vi "FXP Read base - CAR 397265.vi"(8 "error in (no error)":errorcluster, 9 "data in":dbl, 10 "integersize":i32, 11 "shared variable refnum in":refnum<k21>) -> (0 "error out":errorcluster, 1 "data out":dbl, 3 "shared variable refnum out":refnum<k21>)   [LabVIEW 2020]
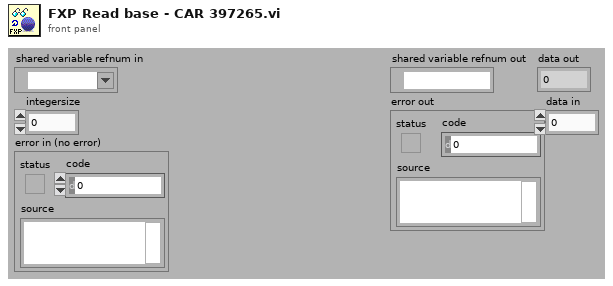
[diagram p1: front panel]
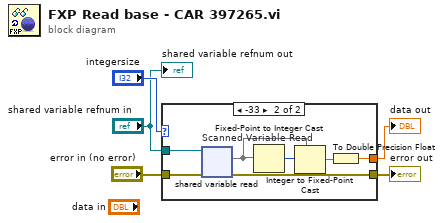
[diagram p0: block diagram]
diagram:
  n1 = case shown="-33" "integersize" {
    tunnel: "error in (no error)" -> [w6 w13]
    tunnel: [w6 w12] -> w3
    tunnel: "shared variable refnum in" -> [_ w11]
    tunnel: [_ w10] -> w1
    frame 2048, Default {
    }
    frame -33 {
      n2 = shared-variable-read "Scanned Variable Read"(w11, w13) -> (w12:errorcluster, w7)  [unwired: 1 in, 2 out]
      n3 = Fixed-Point to Integer Cast(1:w7) -> (0:w8:i32)
      n4 = Integer to Fixed-Point Cast(fixed-point type=w7, integer=w8) -> (fixed-point=w9:fxp<+/-,32,32>)
      n5 = To Double Precision Float(number=w9) -> (double precision float=w10:dbl)
    }
  }
  "error out" <- w3
  "data out" <- w1
  "shared variable refnum out" <- "shared variable refnum in"
